vi "Digital Input.vi"(11 "DIO Channel":T1=enum."DIO MXP 0") -> ()   [LabVIEW 2025]
uses:
  <vilib>/Rock Robotics/SystemInterfaces/DIO/FPGA_DIOChannel.ctl
panel:
  out "DI Status":bool
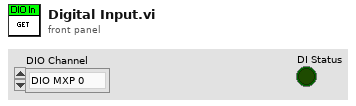
[diagram p1: front panel]
types:
  T1 = typedef "FPGA_DIOChannel.ctl" = enum8{"DIO 0", "DIO 1", "DIO 2", "DIO 3", "DIO 4", "DIO 5", "DIO 6", "DIO 7", "DIO 8", "DIO 9", "DIO MXP 0", "DIO MXP 1", "DIO MXP 2", "DIO MXP 3", "DIO MXP 4", "DIO MXP 5", "DIO MXP 6", "DIO MXP 7", "DIO MXP 8", "DIO MXP 9", "DIO MXP 10", "DIO MXP 11", "DIO MXP 12", "DIO MXP 13", "DIO MXP 14", "DIO MXP 15", "SPI Port CS1", "SPI Port CS2", "SPI Port CS3", "SPI Port MISO", "SPI Port MOSI", "Invalid"}
  T2 = typedef "WPI_DigitalInputDevRef.ctl" = cluster{"DevStatus":errorcluster, "DIO Channel":T1}
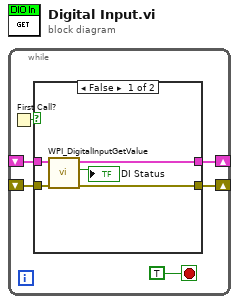
[diagram p0: block diagram]
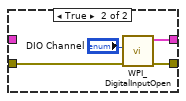
[diagram p2: hidden frame]
diagram:
  n1 = while {
    shift-right: [w3] -> _
    shift-left: _ -> [w4]
    shift-right: [w2] -> _
    shift-left: _ -> [w1]
    stop <- TRUE stop-if-true
    n2 = First Call?() -> (First Call?: T/F=w5:bool)
    n3 = case shown="False" w5 {
      tunnel: w4 -> [w10 w15]
      tunnel: [w8 w14] -> w3
      tunnel: [w9 w13] -> w2
      tunnel: w1 -> [w11 _]
      frame False {
        n4 = call <vilib>:"WPI_DigitalInputGetValue.vi"("error in (no error)"=w10, "DigitalInputDevRef"=w11) -> ("error out"=w8:errorcluster, "Value"=→"DI Status":bool, "DigitalInputDevRef"=w9:T2)  [unwired: 7 in]
      }
      frame True {
        n5 = call <vilib>:"WPI_DigitalInputOpen.vi"("error in (no error)"=w15, "DIO Channel"="DIO Channel") -> ("error out"=w14:errorcluster, "DigitalInputDevRef"=w13:T2)  [unwired: 8 in]
      }
    }
  }
